vi "LEP_RV_BuildSpec_ApplicationInfoDlg.vi"(8 "error in (no error)":errorcluster, 10 "page sync rendezvous":T3, 11 "Close Event":refnum<user-event>) -> ()   [LabVIEW 2011]
doc: "Defines the build options for the application."
uses:
  resource/dialog/PreferencesDialog/optionsFrame_EventData1.ctl
  resource/dialog/PreferencesDialog/optionsFrame_PageInitData.ctl
  <vilib>/Platform/EmbProject/Plugins/utilities/LEP_Utilities_GetSetProjectData_Variant.vi
  <vilib>/Platform/EmbProject/Plugins/utilities/LEP_Utilities_GetSetProjectData_U32.vi
panel:
  in  "Build Specification ID":string caption="BuildSpecificatio ID"
  out "Build settings conflicts":i32(listbox)=-1
  in  "Constant deallocation":u16(ring) caption="Deallocate constants" items=["Out of scope", "VI end", "Application end"]
  in  "Constant allocation":u16(ring) caption="Allocate constants" items=["First use", "Containing Loop", "VI initialization", "Application initialization"]
  in  "Run-Time Options":u16(ring) items=["No optimizations", "Optimize for speed", "Optimize for size", "Custom..."]
  in  "Enable debugging":bool caption="Enable debugging\nCurrent debug mode: JTAG"
  in  "ExpressionFolding":bool caption="Enable expression folding"
  in  "Debug options":T1(radio)
  in  "Build specification name":string
  in  "Generate C function calls":bool
  in  "Generate integer only":bool
  in  "Use stack variables":bool
  in  "Disable parallel execution":bool
  in  "Generate guard code":bool
  in  "Page VI Init Data":T2
  in  "error msg format string":string="There was a problem applying the options from the %s category. The error message is \"%s.\""
  # "Execution Location"
  # "Execution Behavior"
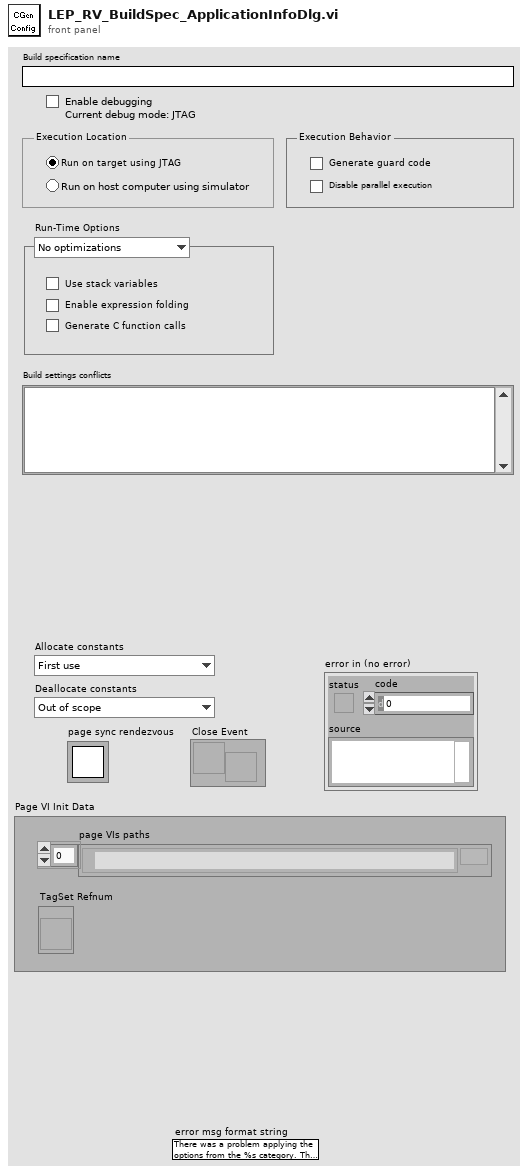
[diagram p1: front panel]
types:
  T1 = enum32{"Run on target using JTAG", "Run on host computer using simulator"}
  T2 = typedef "optionsFrame_PageInitData.ctl" = cluster{"page VIs paths":path[], "TagSet Refnum":refnum<vi>}
  T3 = typedef "Rendezvous RefNum" = refnum<k1>
  T4 = cluster{"Value":bool, "Value":bool, "Value":bool}
  T5 = cluster{"NewVal":bool, "Value":bool, "Value":bool}
  T6 = cluster{"Value":bool, "NewVal":bool, "Value":bool}
  T7 = cluster{"Value":bool, "Value":bool, "NewVal":bool}
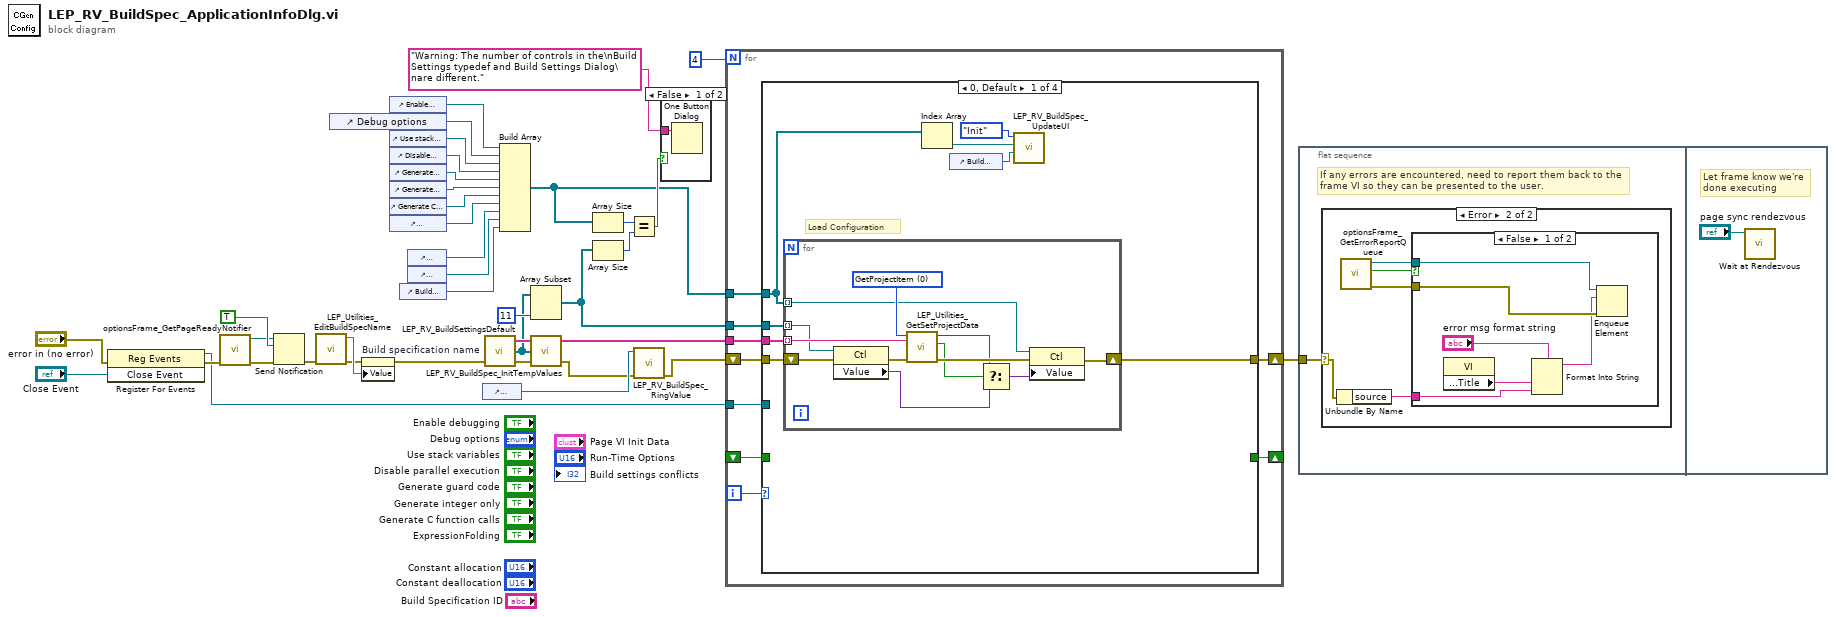
[diagram p0: block diagram]
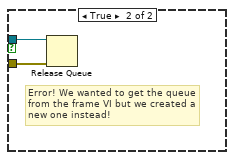
[diagram p3: hidden frame]
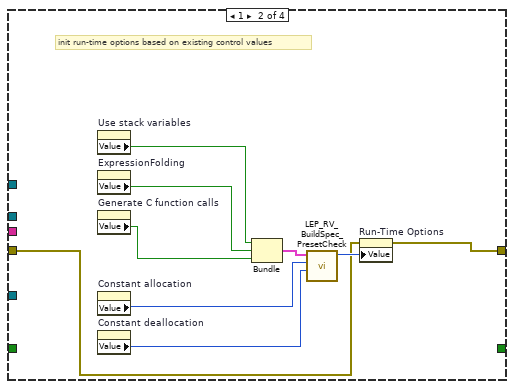
[diagram p5: hidden frame]
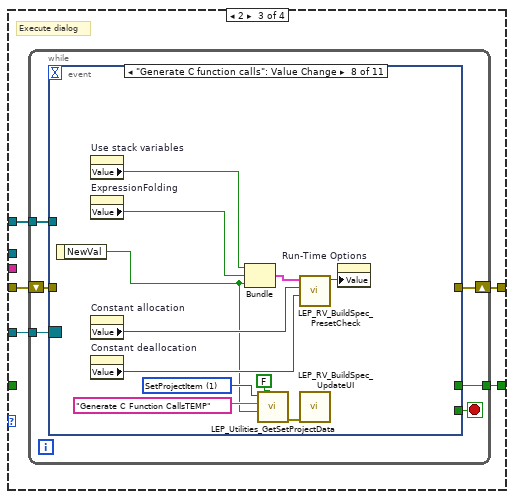
[diagram p6: hidden frame]
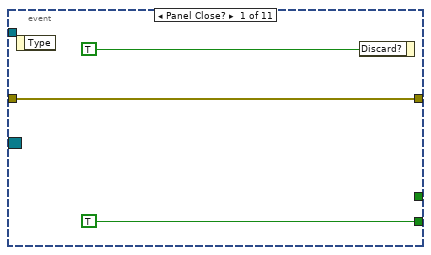
[diagram p7: hidden frame]
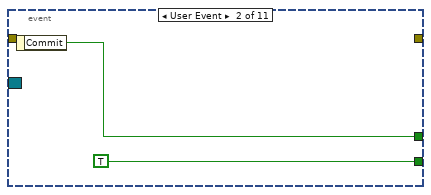
[diagram p8: hidden frame]
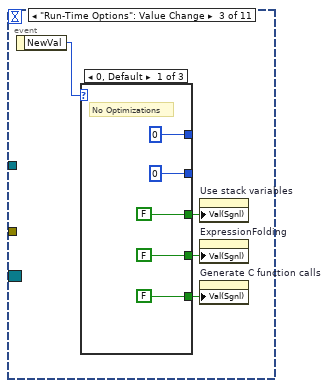
[diagram p9: hidden frame]
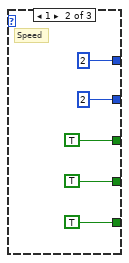
[diagram p10: hidden frame]
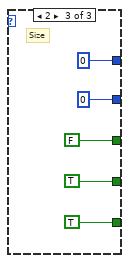
[diagram p11: hidden frame]
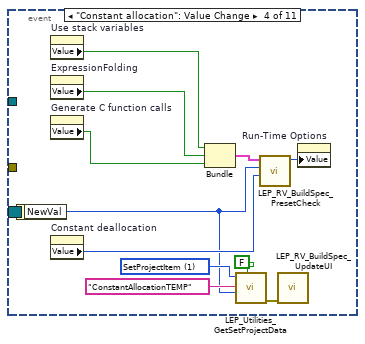
[diagram p12: hidden frame]
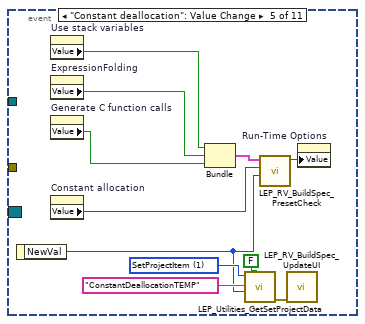
[diagram p13: hidden frame]
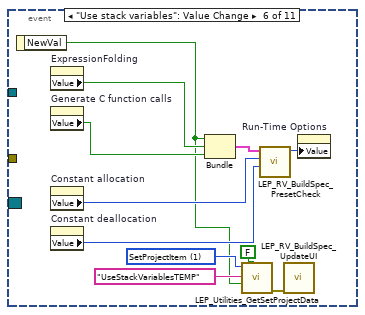
[diagram p14: hidden frame]
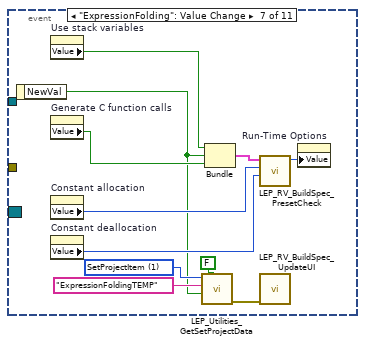
[diagram p15: hidden frame]
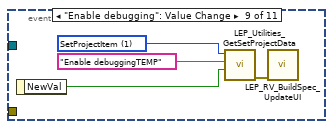
[diagram p16: hidden frame]
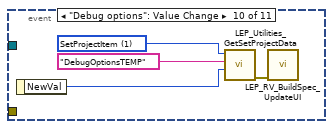
[diagram p17: hidden frame]
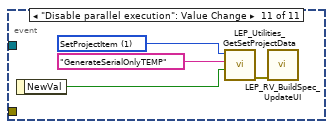
[diagram p18: hidden frame]
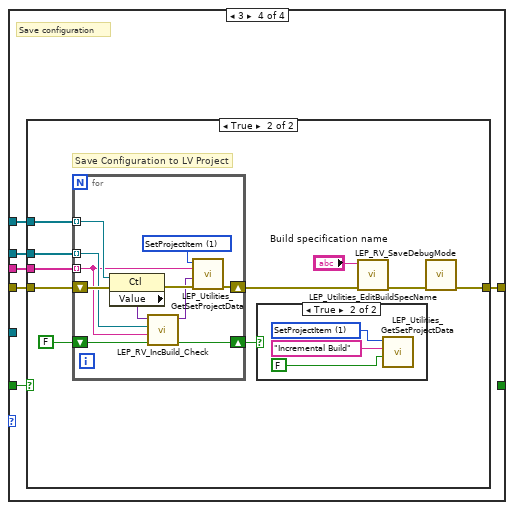
[diagram p19: hidden frame]
diagram:
  n1 = register-events(error in="error in (no error)", "Close Event") -> (reference out=w23:refnum<event-registration>, error out=w25:errorcluster)  [unwired: 1 in]
  n2 = call "optionsFrame_GetPageReadyNotifier.vi"("error in (no error)"=w25) -> ("error out"=w24:errorcluster, "notifier out"=w26:refnum<notifier>)  [unwired: 9 out]
  n3 = Send Notification(notification=TRUE, notifier=w26, error in (no error)=w24) -> (error out=w19:errorcluster)  [unwired: 1 out]
  n4 = call <vilib>:"LEP_Utilities_EditBuildSpecName.vi"("error in"=w19) -> ("error out"=w17:errorcluster, "build spec name"=w18:string)  [unwired: 1 in, 8 out]
  n5 = control-ref of="Debug options"() -> (w14:refnum<vi>)
  n6 = property on="Build specification name" class="Str"(error in=w17, "Value"=w18) -> (error out=w16:errorcluster)  [unwired: 1 in, 1 out]
  n7 = control-ref of="Enable debugging"() -> (w13:refnum<vi>)
  n8 = control-ref of="Use stack variables"() -> (w21:refnum<vi>)
  n9 = control-ref of="Disable parallel execution"() -> (w37:refnum<vi>)
  n10 = control-ref of="Generate guard code"() -> (w36:refnum<vi>)
  n11 = control-ref of="Generate integer only"() -> (w35:refnum<vi>)
  n12 = control-ref of="Generate C function calls"() -> (w34:refnum<vi>)
  n13 = control-ref of="ExpressionFolding"() -> (w20:refnum<vi>)
  n14 = control-ref of="Build Specification ID"() -> (w4:refnum<vi>)
  n15 = control-ref of="Constant allocation"() -> (w8:refnum<vi>)
  n16 = control-ref of="Constant deallocation"() -> (w9:refnum<vi>)
  n17 = control-ref of="Run-Time Options"() -> (w7:refnum<vi>)
  n18 = call "LEP_RV_BuildSettingsDefault.vi"("error in (no error)"=w16) -> ("error out"=w12:errorcluster, "Default Values"=w2:refnum<vi>[], "Attribute Name"=w11:string[])  [unwired: 2 out]
  n19 = Build Array(w13, w14, w21, w37, w36, w35, w34, w20, w8, w9, w4) -> (w31:refnum<vi>[])
  n20 = Array Subset(array=w2, length=11) -> (w1:refnum<vi>[])  [unwired: 1 in]
  n21 = call "LEP_RV_BuildSpec_InitTempValues.vi"("error in (no error)"=w12, "Default Values"=w2, "Attribute Name"=w11) -> ("error out"=w6:errorcluster, "Attribute Name"=w10:string[])  [unwired: 1 out]
  n22 = Array Size(array=w31) -> (size(s)=w33:i32)
  n23 = Array Size(array=w1) -> (size(s)=w15:i32)
  n24 = Equal?(x=w33, y=w15) -> (x = y?=w32:bool)
  n25 = call "LEP_RV_BuildSpec_RingValue.vi"("error in (no error)"=w6, "Ring Refnum"=w7) -> ("error out"=w5:errorcluster)  [unwired: 9 out]
  n26 = case shown="False" w32 {
    tunnel: "Warning: The number of controls in the\nBuild Settings typedef and Build Settings Dialog\nare different." -> [w39 _]
    frame False {
      n27 = One Button Dialog(message=w39) -> ()  [unwired: 2 out]
    }
    frame True {
    }
  }
  n28 = for {
    N: 4 -> [_]
    shift-right: [w46] -> w22
    shift-left: w5 -> [w47]
    shift-right: [w45] -> _
    shift-left: _ -> [w44]
    tunnel: w31 -> [w43]
    tunnel: w10 -> [w42]
    tunnel: w1 -> [w41]
    tunnel: w23 -> [w40]
    i -> [w48]
    n29 = case shown="0, Default" w48 {
      tunnel: w47 -> [w56 w70 w82 w184]
      tunnel: [w53 w69 w81 w183] -> w46
      tunnel: [_ _ w80 _] -> w45
      tunnel: w44 -> [_ _ _ w185]
      tunnel: w43 -> [w52 _ w79 w181]
      tunnel: w42 -> [w55 _ _ w182]
      tunnel: w41 -> [w54 _ _ w180]
      tunnel: w40 -> [_ _ w78 _]
      frame 0, Default {
        # "Load Configuration"
        n30 = for {
          tunnel: w52 -> [w67] mode=indexing
          shift-right: [w65] -> w53
          shift-left: w56 -> [w63]
          tunnel: w55 -> [w64] mode=indexing
          tunnel: w54 -> [w61] mode=indexing
          w68 = u16 0 items=["GetProjectItem", "SetProjectItem"] ("Command")
          n31 = property class="Ctl"(reference=w61, error in=w63) -> (error out=w62:errorcluster, "Value"=w57:variant)  [unwired: 1 out]
          n32 = call-poly <vilib>:"LEP_Utilities_GetSetProjectData.vi"("error in"=w62, "ItemName"=w64, "Command"=w68) -> ("error out"=w66:errorcluster, "Found/Replaced?"=w58:bool, "Variant Out"=w59:variant)  [unwired: 2 in, 4 out]
          n33 = Select(t=w59, s=w58, f=w57) -> (s? t:f=w60:variant)
          n34 = property class="Ctl"(reference=w67, error in=w66, "Value"=w60) -> (error out=w65:errorcluster)  [unwired: 1 out]
        }
        n35 = Index Array(array=w52) -> (element=w50:refnum<vi>)  [unwired: 1 in]
        n36 = control-ref of="Build settings conflicts"() -> (w49:refnum<vi>)
        n37 = call "LEP_RV_BuildSpec_UpdateUI.vi"("Build conflicts ref"=w49, "Enable debugging ref"=w50, "Action"=enum16{"Init", "UpdateUI"}."Init" ("Enum")) -> ()  [unwired: 1 in, 8 out]
      }
      frame 1 {
        # "init run-time options based on existing control values"
        n38 = property on="Use stack variables" class="Bool (strict)"() -> ("Value"=w77:bool)  [unwired: 2 in, 2 out]
        n39 = property on="ExpressionFolding" class="Bool (strict)"() -> ("Value"=w76:bool)  [unwired: 2 in, 2 out]
        n40 = property on="Generate C function calls" class="Bool (strict)"() -> ("Value"=w75:bool)  [unwired: 2 in, 2 out]
        n41 = property on="Constant allocation" class="Ring (strict)"() -> ("Value"=w71:u16)  [unwired: 2 in, 2 out]
        n42 = property on="Constant deallocation" class="Ring (strict)"() -> ("Value"=w73:u16)  [unwired: 2 in, 2 out]
        n43 = Bundle("Value"=w77, "Value"=w76, "Value"=w75) -> (w74:T4)  [unwired: 1 out]
        n44 = call "LEP_RV_BuildSpec_PresetCheck.vi"("Constant deallocation"=w73, "Constant allocation"=w71, "Code generation options"=w74) -> ("Run-Time Options"=w72:u16)  [unwired: 8 out]
        n45 = property on="Run-Time Options" class="Ring (strict)"(error in=w70, "Value"=w72) -> (error out=w69:errorcluster)  [unwired: 1 in, 1 out]
      }
      frame 2 {
        # "Execute dialog"
        n46 = while {
          shift-right: [w87] -> w81
          shift-left: w82 -> [w88]
          tunnel: [w86] -> w80
          tunnel: w79 -> [w84]
          tunnel: w78 -> [w83]
          stop <- w85 stop-if-true
          n47 = event shown="[7] \"Generate C function calls\": Value Change" {
            selector: w83 -> [_ _ _ _ _ _ _ _ _ _ _]
            dyn-events: _ -> [_ _ _ _ _ _ _ _ _ _ _]
            timeout: _ -> [_ _ _ _ _ _ _ _ _ _ _]
            tunnel: w88 -> [w90 _ _ _ _ _ _ _ _ _ _]
            tunnel: [w90 _ _ _ _ _ _ _ _ _ _] -> w87
            tunnel: [_ w92 _ _ _ _ _ _ _ _ _] -> w86
            tunnel: [TRUE TRUE ("Cancel") _ _ _ _ _ _ _ _ _] -> w85
            tunnel: w84 -> [_ _ _ _ _ _ _ _ _ _ _]
            event Panel Close? {
              n48 = event-data() -> ()  [unwired: 2 out]
              n49 = event-data("Discard?"=TRUE) -> ()  [unwired: 1 in, 1 out]
            }
            event User Event {
              n50 = event-data() -> ("Commit"=w92:bool)  [unwired: 1 out]
            }
            event "Run-Time Options": Value Change {
              n51 = event-data() -> ("NewVal"=w97:u16)  [unwired: 1 out]
              n52 = case shown="0, Default" w97 {
                tunnel: [u16 0 ("Value (Signaling)") u16 2 ("Value (Signaling)") u16 0 ("Value (Signaling)")] -> _
                tunnel: [u16 0 ("Value (Signaling)") u16 2 ("Value (Signaling)") u16 0 ("Value (Signaling)")] -> _
                tunnel: [FALSE TRUE FALSE] -> w95
                tunnel: [FALSE TRUE TRUE] -> w96
                tunnel: [FALSE TRUE TRUE] -> w94
                frame 0, Default {
                  # "No Optimizations"
                }
                frame 1 {
                  # "Speed"
                }
                frame 2 {
                  # "Size"
                }
              }
              n53 = property on="Use stack variables" class="Bool (strict)"("Val(Sgnl)"=w95) -> ()  [unwired: 2 in, 2 out]
              n54 = property on="ExpressionFolding" class="Bool (strict)"("Val(Sgnl)"=w96) -> ()  [unwired: 2 in, 2 out]
              n55 = property on="Generate C function calls" class="Bool (strict)"("Val(Sgnl)"=w94) -> ()  [unwired: 2 in, 2 out]
            }
            event "Constant allocation": Value Change {
              w116 = u16 1 items=["GetProjectItem", "SetProjectItem"] ("Command")
              n56 = event-data() -> ("NewVal"=w113:u16)  [unwired: 1 out]
              n57 = property on="Use stack variables" class="Bool (strict)"() -> ("Value"=w123:bool)  [unwired: 2 in, 2 out]
              n58 = property on="ExpressionFolding" class="Bool (strict)"() -> ("Value"=w122:bool)  [unwired: 2 in, 2 out]
              n59 = property on="Generate C function calls" class="Bool (strict)"() -> ("Value"=w121:bool)  [unwired: 2 in, 2 out]
              n60 = property on="Constant deallocation" class="Ring (strict)"() -> ("Value"=w119:u16)  [unwired: 2 in, 2 out]
              n61 = Bundle("Value"=w123, "Value"=w122, "Value"=w121) -> (w120:T4)  [unwired: 1 out]
              n62 = call-poly <vilib>:"LEP_Utilities_GetSetProjectData.vi"("Is Persistent"=FALSE, "data in"=w113, "ItemName"="ConstantAllocationTEMP", "Command"=w116) -> ("error out"=w117:errorcluster)  [unwired: 2 in, 5 out]
              n63 = call "LEP_RV_BuildSpec_PresetCheck.vi"("Constant deallocation"=w119, "Constant allocation"=w113, "Code generation options"=w120) -> ("Run-Time Options"=w118:u16)  [unwired: 8 out]
              n64 = call "LEP_RV_BuildSpec_UpdateUI.vi"("error in (no error)"=w117) -> ()  [unwired: 3 in, 8 out]
              n65 = property on="Run-Time Options" class="Ring (strict)"("Value"=w118) -> ()  [unwired: 2 in, 2 out]
            }
            event "Constant deallocation": Value Change {
              w127 = u16 1 items=["GetProjectItem", "SetProjectItem"] ("Command")
              n66 = event-data() -> ("NewVal"=w124:u16)  [unwired: 1 out]
              n67 = property on="Use stack variables" class="Bool (strict)"() -> ("Value"=w134:bool)  [unwired: 2 in, 2 out]
              n68 = property on="ExpressionFolding" class="Bool (strict)"() -> ("Value"=w133:bool)  [unwired: 2 in, 2 out]
              n69 = property on="Generate C function calls" class="Bool (strict)"() -> ("Value"=w132:bool)  [unwired: 2 in, 2 out]
              n70 = property on="Constant allocation" class="Ring (strict)"() -> ("Value"=w130:u16)  [unwired: 2 in, 2 out]
              n71 = Bundle("Value"=w134, "Value"=w133, "Value"=w132) -> (w131:T4)  [unwired: 1 out]
              n72 = call-poly <vilib>:"LEP_Utilities_GetSetProjectData.vi"("Is Persistent"=FALSE, "data in"=w124, "ItemName"="ConstantDeallocationTEMP", "Command"=w127) -> ("error out"=w128:errorcluster)  [unwired: 2 in, 5 out]
              n73 = call "LEP_RV_BuildSpec_PresetCheck.vi"("Constant deallocation"=w124, "Constant allocation"=w130, "Code generation options"=w131) -> ("Run-Time Options"=w129:u16)  [unwired: 8 out]
              n74 = call "LEP_RV_BuildSpec_UpdateUI.vi"("error in (no error)"=w128) -> ()  [unwired: 3 in, 8 out]
              n75 = property on="Run-Time Options" class="Ring (strict)"("Value"=w129) -> ()  [unwired: 2 in, 2 out]
            }
            event "Use stack variables": Value Change {
              w139 = u16 1 items=["GetProjectItem", "SetProjectItem"] ("Command")
              n76 = event-data() -> ("NewVal"=w135:bool)  [unwired: 1 out]
              n77 = property on="ExpressionFolding" class="Bool (strict)"() -> ("Value"=w145:bool)  [unwired: 2 in, 2 out]
              n78 = property on="Generate C function calls" class="Bool (strict)"() -> ("Value"=w144:bool)  [unwired: 2 in, 2 out]
              n79 = property on="Constant allocation" class="Ring (strict)"() -> ("Value"=w142:u16)  [unwired: 2 in, 2 out]
              n80 = property on="Constant deallocation" class="Ring (strict)"() -> ("Value"=w136:u16)  [unwired: 2 in, 2 out]
              n81 = Bundle("NewVal"=w135, "Value"=w145, "Value"=w144) -> (w143:T5)  [unwired: 1 out]
              n82 = call-poly <vilib>:"LEP_Utilities_GetSetProjectData.vi"("Is Persistent"=FALSE, "Variant In"=w135, "ItemName"="UseStackVariablesTEMP", "Command"=w139) -> ("error out"=w140:errorcluster)  [unwired: 2 in, 5 out]
              n83 = call "LEP_RV_BuildSpec_PresetCheck.vi"("Constant deallocation"=w136, "Constant allocation"=w142, "Code generation options"=w143) -> ("Run-Time Options"=w141:u16)  [unwired: 8 out]
              n84 = call "LEP_RV_BuildSpec_UpdateUI.vi"("error in (no error)"=w140) -> ()  [unwired: 3 in, 8 out]
              n85 = property on="Run-Time Options" class="Ring (strict)"("Value"=w141) -> ()  [unwired: 2 in, 2 out]
            }
            event "ExpressionFolding": Value Change {
              w149 = u16 1 items=["GetProjectItem", "SetProjectItem"] ("Command")
              n86 = event-data() -> ("NewVal"=w147:bool)  [unwired: 1 out]
              n87 = property on="Use stack variables" class="Bool (strict)"() -> ("Value"=w156:bool)  [unwired: 2 in, 2 out]
              n88 = property on="Generate C function calls" class="Bool (strict)"() -> ("Value"=w155:bool)  [unwired: 2 in, 2 out]
              n89 = property on="Constant allocation" class="Ring (strict)"() -> ("Value"=w153:u16)  [unwired: 2 in, 2 out]
              n90 = property on="Constant deallocation" class="Ring (strict)"() -> ("Value"=w152:u16)  [unwired: 2 in, 2 out]
              n91 = call-poly <vilib>:"LEP_Utilities_GetSetProjectData.vi"("Is Persistent"=FALSE, "Variant In"=w147, "ItemName"="ExpressionFoldingTEMP", "Command"=w149) -> ("error out"=w146:errorcluster)  [unwired: 2 in, 5 out]
              n92 = Bundle("Value"=w156, "NewVal"=w147, "Value"=w155) -> (w154:T6)  [unwired: 1 out]
              n93 = call "LEP_RV_BuildSpec_PresetCheck.vi"("Constant deallocation"=w152, "Constant allocation"=w153, "Code generation options"=w154) -> ("Run-Time Options"=w151:u16)  [unwired: 8 out]
              n94 = call "LEP_RV_BuildSpec_UpdateUI.vi"("error in (no error)"=w146) -> ()  [unwired: 3 in, 8 out]
              n95 = property on="Run-Time Options" class="Ring (strict)"("Value"=w151) -> ()  [unwired: 2 in, 2 out]
            }
            event "Generate C function calls": Value Change {
              w161 = u16 1 items=["GetProjectItem", "SetProjectItem"] ("Command")
              n96 = event-data() -> ("NewVal"=w159:bool)  [unwired: 1 out]
              n97 = property on="Use stack variables" class="Bool (strict)"() -> ("Value"=w167:bool)  [unwired: 2 in, 2 out]
              n98 = property on="ExpressionFolding" class="Bool (strict)"() -> ("Value"=w166:bool)  [unwired: 2 in, 2 out]
              n99 = property on="Constant allocation" class="Ring (strict)"() -> ("Value"=w165:u16)  [unwired: 2 in, 2 out]
              n100 = property on="Constant deallocation" class="Ring (strict)"() -> ("Value"=w164:u16)  [unwired: 2 in, 2 out]
              n101 = Bundle("Value"=w167, "Value"=w166, "NewVal"=w159) -> (w157:T7)  [unwired: 1 out]
              n102 = call-poly <vilib>:"LEP_Utilities_GetSetProjectData.vi"("Is Persistent"=FALSE, "Variant In"=w159, "ItemName"="Generate C Function CallsTEMP", "Command"=w161) -> ("error out"=w158:errorcluster)  [unwired: 2 in, 5 out]
              n103 = call "LEP_RV_BuildSpec_PresetCheck.vi"("Constant deallocation"=w164, "Constant allocation"=w165, "Code generation options"=w157) -> ("Run-Time Options"=w163:u16)  [unwired: 8 out]
              n104 = call "LEP_RV_BuildSpec_UpdateUI.vi"("error in (no error)"=w158) -> ()  [unwired: 3 in, 8 out]
              n105 = property on="Run-Time Options" class="Ring (strict)"("Value"=w163) -> ()  [unwired: 2 in, 2 out]
            }
            event "Enable debugging": Value Change {
              w171 = u16 1 items=["GetProjectItem", "SetProjectItem"] ("Command")
              n106 = event-data() -> ("NewVal"=w169:bool)  [unwired: 1 out]
              n107 = call-poly <vilib>:"LEP_Utilities_GetSetProjectData.vi"("Variant In"=w169, "ItemName"="Enable debuggingTEMP", "Command"=w171) -> ("error out"=w168:errorcluster)  [unwired: 2 in, 6 out]
              n108 = call "LEP_RV_BuildSpec_UpdateUI.vi"("error in (no error)"=w168) -> ()  [unwired: 3 in, 8 out]
            }
            event "Debug options": Value Change {
              w175 = u16 1 items=["GetProjectItem", "SetProjectItem"] ("Command")
              n109 = event-data() -> ("NewVal"=w173:T1)  [unwired: 1 out]
              n110 = call-poly <vilib>:"LEP_Utilities_GetSetProjectData.vi"("data in"=w173, "ItemName"="DebugOptionsTEMP", "Command"=w175) -> ("error out"=w172:errorcluster)  [unwired: 2 in, 6 out]
              n111 = call "LEP_RV_BuildSpec_UpdateUI.vi"("error in (no error)"=w172) -> ()  [unwired: 3 in, 8 out]
            }
            event "Disable parallel execution": Value Change {
              w179 = u16 1 items=["GetProjectItem", "SetProjectItem"] ("Command")
              n112 = event-data() -> ("NewVal"=w177:bool)  [unwired: 1 out]
              n113 = call-poly <vilib>:"LEP_Utilities_GetSetProjectData.vi"("Variant In"=w177, "ItemName"="GenerateSerialOnlyTEMP", "Command"=w179) -> ("error out"=w176:errorcluster)  [unwired: 2 in, 6 out]
              n114 = call "LEP_RV_BuildSpec_UpdateUI.vi"("error in (no error)"=w176) -> ()  [unwired: 3 in, 8 out]
            }
          }
        }
      }
      frame 3 {
        # "Save configuration"
        n115 = case shown="True" w185 {
          tunnel: w184 -> [w186 w196]
          tunnel: [w186 w187] -> w183
          tunnel: w182 -> [_ w195]
          tunnel: w181 -> [_ w194]
          tunnel: w180 -> [_ w190]
          frame False {
          }
          frame True {
            # "Save Configuration to LV Project"
            n116 = for {
              shift-right: [w207] -> w192
              shift-left: w196 -> [w209]
              tunnel: w195 -> [w202] mode=indexing
              tunnel: w194 -> [w204] mode=indexing
              shift-right: [w205] -> w189
              shift-left: FALSE -> [w206]
              tunnel: w190 -> [w203] mode=indexing
              w210 = u16 1 items=["GetProjectItem", "SetProjectItem"] ("Command")
              n117 = property class="Ctl"(reference=w204, error in=w209) -> (error out=w208:errorcluster, "Value"=w201:variant)  [unwired: 1 out]
              n118 = call "LEP_RV_IncBuild_Check.vi"("changed?"=w206, "attribute name"=w202, "default value"=w203, "control value"=w201) -> ("changed?"=w205:bool, "control value out"=w200:variant)  [unwired: 6 out]
              n119 = call-poly <vilib>:"LEP_Utilities_GetSetProjectData.vi"("error in"=w208, "Variant In"=w200, "ItemName"=w202, "Command"=w210) -> ("error out"=w207:errorcluster)  [unwired: 1 in, 6 out]
            }
            n120 = case shown="True" w189 {
              frame False {
              }
              frame True {
                w199 = u16 1 items=["GetProjectItem", "SetProjectItem"] ("Command")
                n121 = call-poly <vilib>:"LEP_Utilities_GetSetProjectData.vi"("Variant In"=FALSE, "ItemName"="Incremental Build", "Command"=w199) -> ()  [unwired: 2 in, 7 out]
              }
            }
            n122 = call <vilib>:"LEP_Utilities_EditBuildSpecName.vi"("error in"=w192, "new build spec name"="Build specification name") -> ("error out"=w188:errorcluster)  [unwired: 9 out]
            n123 = call "LEP_RV_SaveDebugMode.vi"("error in"=w188) -> ("error out"=w187:errorcluster)  [unwired: 10 in]
          }
        }
      }
    }
  }
  n124 = flat-sequence {
    tunnel: w22 -> [w211]
    frame #0 {
      # "If any errors are encountered, need to report them back to the \nframe VI so they can be presented to the user."
      n125 = case shown="Error" w211 {
        selector: w211 -> [_ w213]
        frame No Error {
        }
        frame Error {
          n126 = Unbundle By Name(w213) -> ("source"=w212:string)
          n127 = call "optionsFrame_GetErrorReportQueue.vi"() -> ("error out"=w214:errorcluster, "created new?"=w216:bool, "queue out"=w215:refnum<queue>)  [unwired: 9 out]
          n128 = case shown="False" w216 {
            tunnel: w215 -> [w222 w224]
            tunnel: w214 -> [w221 w223]
            tunnel: w212 -> [w218 _]
            frame False {
              n129 = property class="VI"() -> ("Front Panel.Title"=w219:string)  [unwired: 2 in, 2 out]
              n130 = Format Into String(format string="error msg format string", w219, w218) -> (resulting string=w217:string)  [unwired: 2 in, 1 out]
              n131 = Enqueue Element(queue=w222, element=w217, error in (no error)=w221) -> ()  [unwired: 4 out]
            }
            frame True {
              # "Error! We wanted to get the queue\nfrom the frame VI but we created a\nnew one instead!"
              n132 = Release Queue(queue=w224, error in (no error)=w223) -> ()  [unwired: 4 out]
            }
          }
        }
      }
    }
    frame #1 {
      # "Let frame know we're \ndone executing"
      n133 = call <vilib>:"Wait at Rendezvous.vi"("rendezvous"="page sync rendezvous") -> ()  [unwired: 2 in, 5 out]
    }
  }
